vi "LPA400_calculate_checksum.vi"(1 "String":string) -> (0 "Checksum":string)   [LabVIEW 2010]
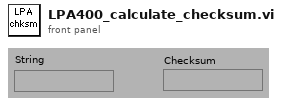
[diagram p1: front panel]
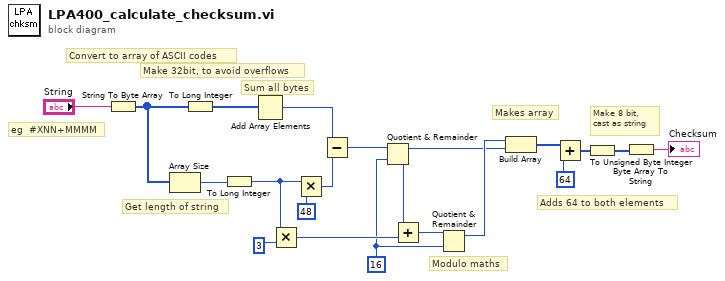
[diagram p0: block diagram]
diagram:
  w2 = 16 ("y")
  # "Modulo maths"
  # "Make 8 bit, cast as string"
  # "Adds 64 to both elements"
  # "Makes array"
  # "Get length of string"
  # "Sum all bytes"
  # "Make 32bit, to avoid overflows"
  # "Convert to array of ASCII codes"
  # "eg  #XNN+MMMM"
  n1 = String To Byte Array(string="String") -> (unsigned byte array=w20:u8[])
  n2 = Array Size(array=w20) -> (size(s)=w19:i32)
  n3 = To Long Integer(number=w20) -> (32bit integer=w18:i32[])
  n4 = To Long Integer(number=w19) -> (32bit integer=w11:i32)
  n5 = Add Array Elements(numeric array=w18) -> (sum=w16:i32)
  n6 = Multiply(x=w11, y=3) -> (x*y=w9:i32)
  n7 = Multiply(x=w11, y=48) -> (x*y=w15:i32)
  n8 = Subtract(x=w16, y=w15) -> (x-y=w14:i32)
  n9 = Quotient & Remainder(x=w14, y=w2) -> (x-y*floor(x/y)=w3:i32, floor(x/y)=w13:i32)
  n10 = Add(x=w13, y=w9) -> (x+y=w8:i32)
  n11 = Quotient & Remainder(x=w8, y=w2) -> (x-y*floor(x/y)=w6:i32)  [unwired: 1 out]
  n12 = Build Array(w6, w3) -> (w5:i32[])
  n13 = Add(x=w5, y=64) -> (x+y=w4:i32[])
  n14 = To Unsigned Byte Integer(number=w4) -> (unsigned 8bit integer=w1:u8[])
  n15 = Byte Array To String(unsigned byte array=w1) -> (string=→"Checksum":string)
